vi "float_unit_conversion.vi"(2 "inverse function (arb. unit to s)?":bool=TRUE, 4 "time":dbl, 5 "time unit":enum16{"s", "ms", "us", "ns"}(ring)) -> (1 "converted time":dbl)   [LabVIEW 2011]
doc: "This VI converts a delay array from seconds to the specified unit."
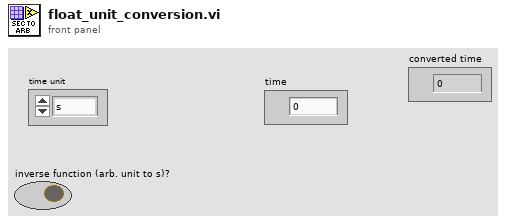
[diagram p1: front panel]
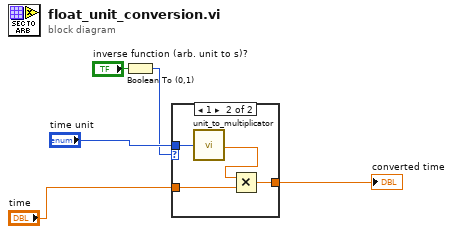
[diagram p0: block diagram]
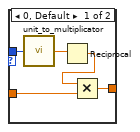
[diagram p2: hidden frame]
diagram:
  n1 = Boolean To (0,1)(Boolean="inverse function (arb. unit to s)?") -> (0, 1=w3:i16)
  n2 = case shown="1" w3 {
    tunnel: "time unit" -> [w10 w14]
    tunnel: [w9 w13] -> w1
    tunnel: "time" -> [w8 w12]
    frame 0, Default {
      n3 = call "unit_to_multiplicator.vi"("time unit"=w10) -> ("multiplicator"=w7:dbl)
      n4 = Reciprocal(x=w7) -> (1/x=w6:dbl)
      n5 = Multiply(x=w6, y=w8) -> (x*y=w9:dbl)
    }
    frame 1 {
      n6 = call "unit_to_multiplicator.vi"("time unit"=w14) -> ("multiplicator"=w11:dbl)
      n7 = Multiply(x=w11, y=w12) -> (x*y=w13:dbl)
    }
  }
  "converted time" <- w1
